vi "Zapisz_INI_AIDI.vi"(7 "Obiekt":string, 8 "error in (no error)":errorcluster, 9 "Kanały cyfrowe":refnum<vi>, 10 "AI Referencje Array":refnum<vi>[](array[refnum]), 11 "configuration file path":path) -> (0 "error out":errorcluster)   [LabVIEW 2014]
doc: "Zapisuje ustawienia kanałów\nanalogowych i cyfrowych do pliku konfiguracyjnego INI"
uses:
  Kontrolki/GUI/DI_aktywacja.ctl
  <vilib>/Utility/config.llb/Write Key (String).vi
  <vilib>/Utility/config.llb/NI_LVConfig.lvlib
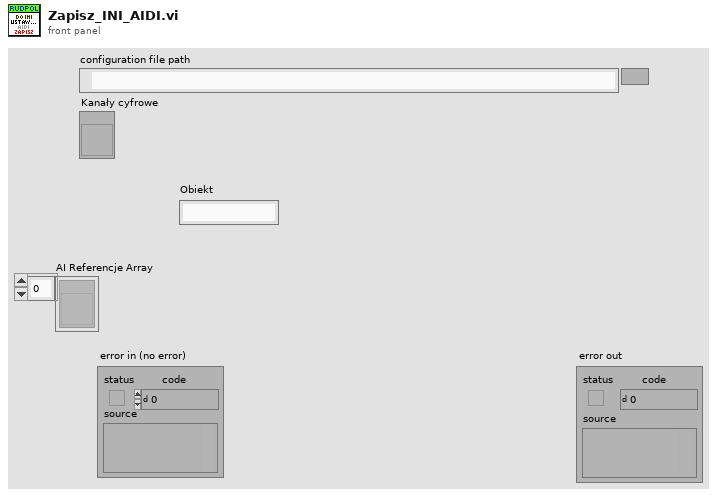
[diagram p1: front panel]
types:
  T1 = typedef "NI_LVConfig.lvlib/Config Data RefNum.ctl" = refnum<k1>
  T2 = typedef "AI_parametry.ctl" = cluster{"Numer":u8, "Opis":string, "Zakres":enum16{"1000V", "300V", "30V", "3V", "0,3V"}, "Filtr":bool, "Typ pomiaru":enum16{"Wartość średnia", "Średnia wyprostowana", "Wartość skuteczna"}, "Aktywny":bool, "Wartość":T3}
  T3 = typedef "AI_wartosc.ctl" = cluster{"X":string, "[ ]":string, "trans X":dbl, "trans U":dbl, "Z tabeli":bool, "Opis":string}
  T4 = enum16{"Wartość średnia", "Średnia wyprostowana", "Wartość skuteczna"}
  T5 = typedef "DI_aktywacja.ctl" = cluster{"DI1":bool, "DI2":bool, "DI3":bool, "DI4":bool, "DI1 Opis":string, "DI2 Opis":string, "DI3 Opis":string, "DI4 Opis":string, "DI1 Amplituda":dbl, "DI2 Amplituda":dbl, "DI3 Amplituda":dbl, "DI4 Amplituda":dbl}
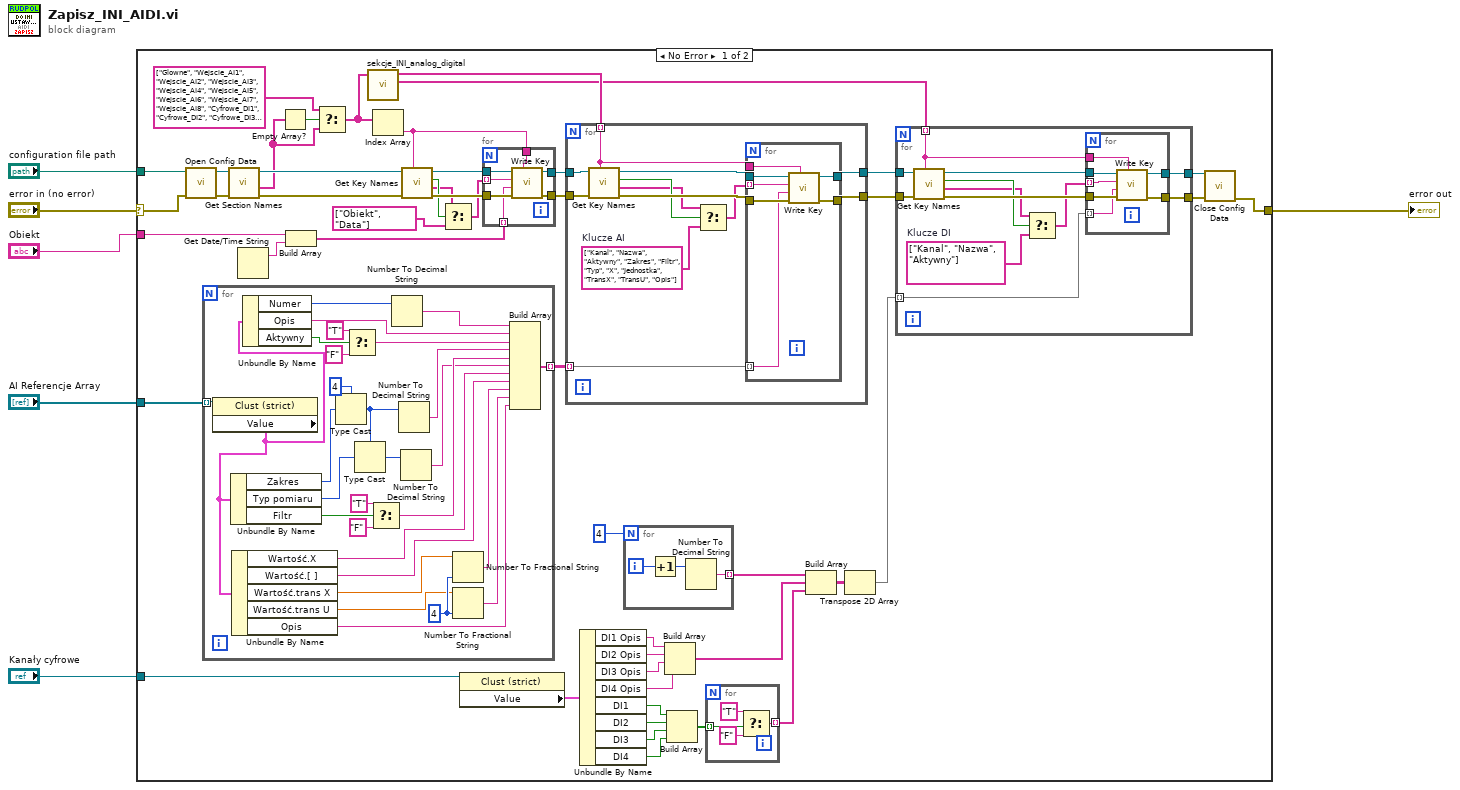
[diagram p0: block diagram]
diagram:
  n1 = case shown="No Error" "error in (no error)" {
    selector: "error in (no error)" -> [w52 w136]
    tunnel: [w31 w136] -> w5
    tunnel: "configuration file path" -> [w51 _]
    tunnel: "Kanały cyfrowe" -> [w41 _]
    tunnel: "AI Referencje Array" -> [w29 _]
    tunnel: "Obiekt" -> [w7 _]
    frame No Error {
      n2 = call <vilib>:"Open Config Data.vi"("error in (no error)"=w52, "configuration file path"=w51) -> ("error out"=w53:errorcluster, "refnum"=w54:T1)  [unwired: 7 in, 1 out]
      n3 = for {
        tunnel: [w106] -> w45 mode=indexing
        tunnel: w29 -> [w81] mode=indexing
        w101 = i16 4 ("precision (6)")
        n4 = property class="Clust (strict)"(reference=w81) -> ("Value"=w82:T2)  [unwired: 1 in, 2 out]
        n5 = Unbundle By Name(w82) -> ("Zakres"=w93:enum16{"1000V", "300V", "30V", "3V", "0,3V"}, "Typ pomiaru"=w87:T4, "Filtr"=w89:bool)
        n6 = Unbundle By Name(w82) -> ("Wartość.X"=w94:string, "Wartość.[ ]"=w95:string, "Wartość.trans X"=w96:dbl, "Wartość.trans U"=w97:dbl, "Opis"=w98:string)
        n7 = Unbundle By Name(w82) -> ("Numer"=w109:u8, "Opis"=w107:string, "Aktywny"=w105:bool)
        n8 = Type Cast(type=u16 4 ("upper limit"), x=w93) -> (*(type *) &x=w86:u16)
        n9 = Select(t="T", s=w105, f="F") -> (s? t:f=w102:string)
        n10 = Type Cast(type=w86, x=w87) -> (*(type *) &x=w84:u16)
        n11 = Select(t="T", s=w89, f="F") -> (s? t:f=w88:string)
        n12 = Number To Decimal String(number=w109) -> (decimal integer string=w108:string)  [unwired: 1 in]
        n13 = Number To Decimal String(number=w86) -> (decimal integer string=w85:string)  [unwired: 1 in]
        n14 = Number To Decimal String(number=w84) -> (decimal integer string=w83:string)  [unwired: 1 in]
        n15 = Number To Fractional String(number=w96, precision (6)=w101) -> (F-format string=w100:string)  [unwired: 2 in]
        n16 = Number To Fractional String(number=w97, precision (6)=w101) -> (F-format string=w99:string)  [unwired: 2 in]
        n17 = Build Array(w108, w107, w102, w85, w88, w83, w94, w95, w100, w99, w98) -> (w106:string[])
      }
      n18 = call <vilib>:"Get Section Names.vi"("error in (no error)"=w53, "refnum"=w54) -> ("error out"=w25:errorcluster, "section names"=w22:string[], "refnum out"=w24:T1)  [unwired: 7 in]
      n19 = Get Date/Time String() -> (date string=w50:string)  [unwired: 3 in, 1 out]
      n20 = Empty Array?(array=w22) -> (empty?=w23:bool)
      n21 = Build Array(w7, w50) -> (w49:string[])
      n22 = Select(t=string[] ["Glowne", "Wejscie_AI1", "Wejscie_AI2", "Wejscie_AI3", "Wejscie_AI4", "Wejscie_AI5", "Wejscie_AI6", "Wejscie_AI7", "Wejscie_AI8", "Cyfrowe_DI1", "Cyfrowe_DI2", "Cyfrowe_DI3", "Cyfrowe_DI4"], s=w23, f=w22) -> (s? t:f=w21:string[])
      n23 = call "sekcje_INI_analog_digital.vi"("section names"=w21) -> ("DI sections"=w44:string[], "AI sections"=w46:string[])  [unwired: 9 in]
      n24 = Index Array(array=w21) -> (element=w26:string)  [unwired: 1 in]
      n25 = call <vilib>:"Get Key Names.vi"("section"=w26, "error in (no error)"=w25, "refnum"=w24) -> ("error out"=w27:errorcluster, "key names"=w18:string[], "section exists?"=w19:bool, "refnum out"=w28:T1)  [unwired: 5 in]
      n26 = Select(t=w18, s=w19, f=string[] ["Obiekt", "Data"]) -> (s? t:f=w17:string[])
      n27 = property class="Clust (strict)"(reference=w41) -> ("Value"=w40:T5)  [unwired: 1 in, 2 out]
      n28 = for {
        tunnel: w26 -> [w135]
        tunnel: w28 -> [w134]
        tunnel: w27 -> [w133]
        tunnel: w17 -> [w132] mode=indexing
        tunnel: w49 -> [w131] mode=indexing
        tunnel: [w130] -> w48
        tunnel: [w129] -> w47
        n29 = call-poly <vilib>:"Write Key.vi"("section"=w135, "error in (no error)"=w133, "value"=w131, "key"=w132, "refnum"=w134) -> ("error out"=w129:errorcluster, "refnum out"=w130:T1)  [unwired: 4 in, 1 out]
      }
      n30 = for {
        tunnel: w48 -> [w121]
        tunnel: w47 -> [w120]
        tunnel: w46 -> [w117] mode=indexing
        tunnel: w45 -> [w116] mode=indexing
        tunnel: [w115] -> w43
        tunnel: [w114] -> w42
        w110 = string[] ["Kanal", "Nazwa", "Aktywny", "Zakres", "Filtr", "Typ", "X", "Jednostka", "TransX", "TransU", "Opis"]  # Klucze AI
        n31 = call <vilib>:"Get Key Names.vi"("section"=w117, "error in (no error)"=w120, "refnum"=w121) -> ("error out"=w119:errorcluster, "key names"=w112:string[], "section exists?"=w113:bool, "refnum out"=w118:T1)  [unwired: 5 in]
        n32 = Select(t=w112, s=w113, f=w110) -> (s? t:f=w111:string[])
        n33 = for {
          tunnel: w119 -> [w126]
          tunnel: w118 -> [w128]
          tunnel: w111 -> [w125] mode=indexing
          tunnel: w117 -> [w127]
          tunnel: w116 -> [w124] mode=indexing
          tunnel: [w123] -> w115
          tunnel: [w122] -> w114
          n34 = call-poly <vilib>:"Write Key.vi"("section"=w127, "error in (no error)"=w126, "value"=w124, "key"=w125, "refnum"=w128) -> ("error out"=w122:errorcluster, "refnum out"=w123:T1)  [unwired: 4 in, 1 out]
        }
      }
      n35 = Unbundle By Name(w40) -> ("DI1 Opis"=w11:string, "DI2 Opis"=w10:string, "DI3 Opis"=w9:string, "DI4 Opis"=w8:string, "DI1"=w14:bool, "DI2"=w15:bool, "DI3"=w13:bool, "DI4"=w12:bool)
      n36 = for {
        N: 4 -> [_]
        tunnel: [w55] -> w38 mode=indexing
        i -> [w57]
        n37 = Increment(x=w57) -> (x+1=w56:i32)
        n38 = Number To Decimal String(number=w56) -> (decimal integer string=w55:string)  [unwired: 1 in]
      }
      n39 = Build Array(w11, w10, w9, w8) -> (w37:string[])
      n40 = Build Array(w14, w15, w13, w12) -> (w39:bool[])
      n41 = for {
        tunnel: w39 -> [w59] mode=indexing
        tunnel: [w58] -> w36 mode=indexing
        n42 = Select(t="T", s=w59, f="F") -> (s? t:f=w58:string)
      }
      n43 = Build Array(w38, w37, w36) -> (w35:string[][])
      n44 = Transpose 2D Array(2D array=w35) -> (transposed array=w34:string[][])
      n45 = for {
        tunnel: w44 -> [w66] mode=indexing
        tunnel: w43 -> [w73]
        tunnel: w42 -> [w72]
        tunnel: w34 -> [w69] mode=indexing
        tunnel: [w68] -> w33
        tunnel: [w67] -> w32
        w65 = string[] ["Kanal", "Nazwa", "Aktywny"]  # Klucze DI
        n46 = call <vilib>:"Get Key Names.vi"("section"=w66, "error in (no error)"=w72, "refnum"=w73) -> ("error out"=w70:errorcluster, "key names"=w63:string[], "section exists?"=w64:bool, "refnum out"=w71:T1)  [unwired: 5 in]
        n47 = Select(t=w63, s=w64, f=w65) -> (s? t:f=w62:string[])
        n48 = for {
          tunnel: w71 -> [w80]
          tunnel: w70 -> [w79]
          tunnel: w62 -> [w78] mode=indexing
          tunnel: w69 -> [w77] mode=indexing
          tunnel: [w76] -> w68
          tunnel: [w75] -> w67
          tunnel: w66 -> [w74]
          n49 = call-poly <vilib>:"Write Key.vi"("section"=w74, "error in (no error)"=w79, "value"=w77, "key"=w78, "refnum"=w80) -> ("error out"=w75:errorcluster, "refnum out"=w76:T1)  [unwired: 4 in, 1 out]
        }
      }
      n50 = call <vilib>:"Close Config Data.vi"("error in (no error)"=w32, "refnum"=w33) -> ("error out"=w31:errorcluster)  [unwired: 8 in, 1 out]
    }
    frame Error {
    }
  }
  "error out" <- w5
